vi "Swap X and Y (single).vi"(8 "error in (no error)":errorcluster, 11 "XY-data":cluster{"X-array":dbl[], "Y-array":dbl[]}) -> (0 "error out":errorcluster, 3 "XY-data out":cluster{"X-array":dbl[], "Y-array":dbl[]} {"Y-array" format="%.2p"; "X-array" format="%.2p"})   [LabVIEW 2019, in "xy_utilities.lvlib"]
doc: "Swap the x and y arrays.\n\nWire data to the data input to determine the polymorphic instance to use or manually select the instance."
uses:
  xy_utilities.lvlib
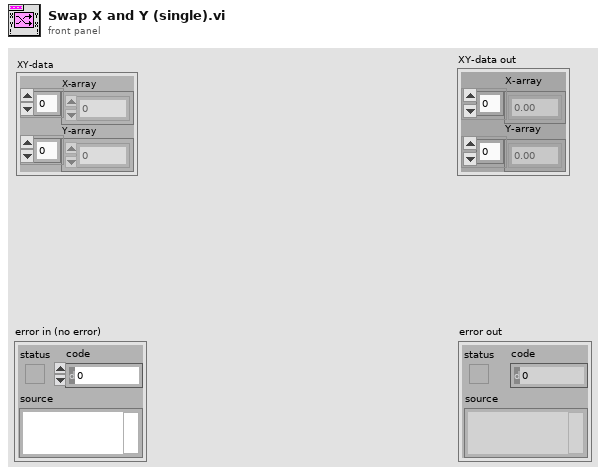
[diagram p1: front panel]
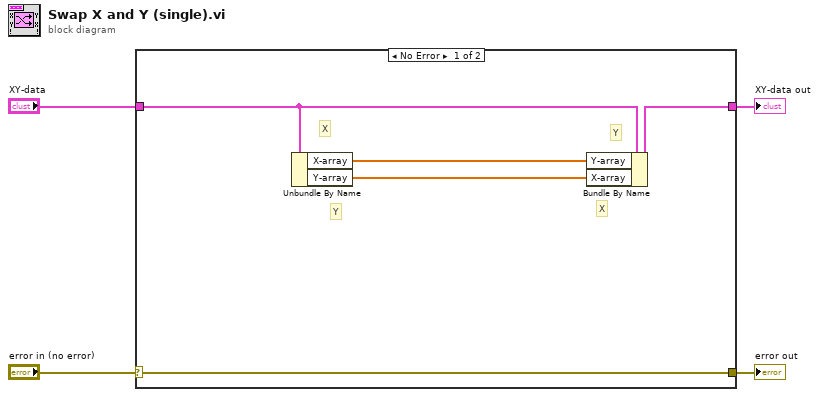
[diagram p0: block diagram]
diagram:
  n1 = case shown="No Error" "error in (no error)" {
    selector: "error in (no error)" -> [w5 w11]
    tunnel: [w5 w11] -> w3
    tunnel: "XY-data" -> [w9 w10]
    tunnel: [w8 w10] -> w1
    frame No Error {
      # "X"
      # "X"
      # "Y"
      # "Y"
      n2 = Unbundle By Name(w9) -> ("X-array"=w7:dbl[], "Y-array"=w6:dbl[])
      n3 = Bundle By Name(cluster=w9, "Y-array"=w7, "X-array"=w6) -> (w8:cluster{"X-array":dbl[], "Y-array":dbl[]})
    }
    frame Error {
    }
  }
  "error out" <- w3
  "XY-data out" <- w1
